vi "Safe Stop IO.vi"(8 "error in":errorcluster, 11 "DAQ Ref Cluster":T1) -> (0 "error out":errorcluster, 3 "DAQ Ref Cluster Out":T1)   [LabVIEW 2021]
uses:
  controls/DAQ Refnums.ctl
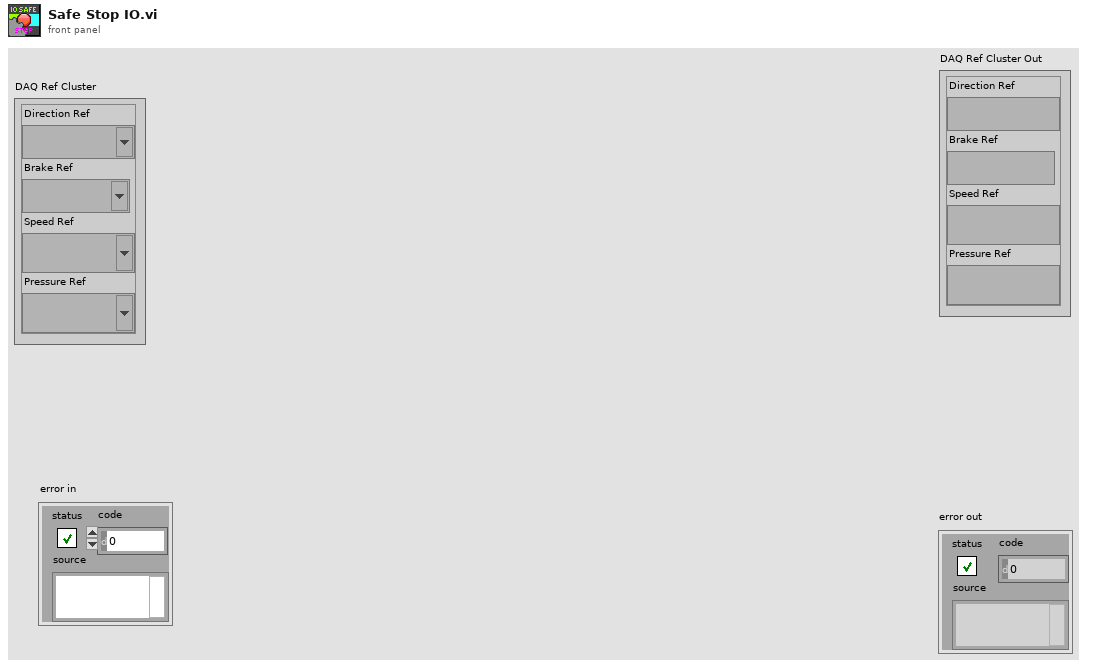
[diagram p1: front panel]
types:
  T1 = typedef "DAQ Refnums.ctl" = cluster{"Direction Ref":refnum<k21>, "Brake Ref":refnum<k21>, "Speed Ref":refnum<k21>, "Pressure Ref":refnum<k21>}
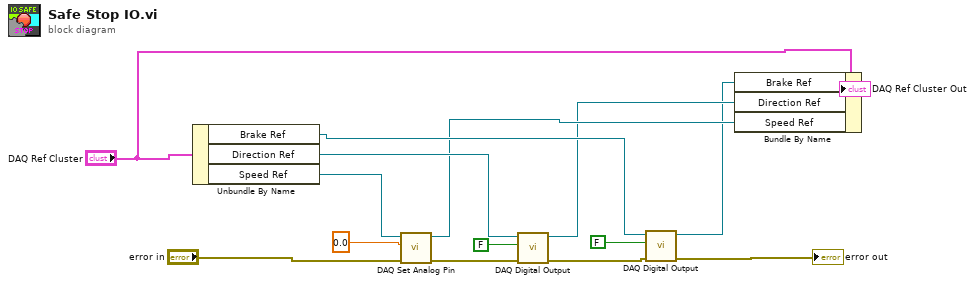
[diagram p0: block diagram]
diagram:
  n1 = Unbundle By Name("DAQ Ref Cluster") -> ("Brake Ref"=w11:refnum<k21>, "Direction Ref"=w12:refnum<k21>, "Speed Ref"=w13:refnum<k21>)
  n2 = call "DAQ Set Analog Pin.vi"("error in"="error in", "Voltage"=0.0, "task/channels in"=w13) -> ("error out"=w5:errorcluster, "task out"=w8:refnum<k21>)  [unwired: 6 in, 1 out]
  n3 = call "DAQ Digital Output.vi"("error in"=w5, "data"=FALSE, "task/channels in"=w12) -> ("error out"=w4:errorcluster, "task out"=w7:refnum<k21>)  [unwired: 6 in, 1 out]
  n4 = call "DAQ Digital Output.vi"("error in"=w4, "data"=FALSE, "task/channels in"=w11) -> ("error out"=→"error out":errorcluster, "task out"=w6:refnum<k21>)  [unwired: 6 in, 1 out]
  n5 = Bundle By Name(cluster="DAQ Ref Cluster", "Brake Ref"=w6, "Direction Ref"=w7, "Speed Ref"=w8) -> (→"DAQ Ref Cluster Out":T1)
